vi "mw-dar.vi"() -> ()   [LabVIEW 2022 SP3]
panel:
  in  "Stopp":bool
  out "Zählung Speicherwerte":dbl
  out "Speichervorgang läuft":bool
  in  "Start Datenspeicherung":bool
  in  "Anzahl Messerte zum speichern":dbl
  out "Maximalwert Kurve 3":dbl format="%#.2g"
  out "Minimalwert Kurve 3":dbl format="%#.2g"
  out "Minimalwert Kurve 2":dbl format="%#.2g"
  out "Maximalwert Kurve 2":dbl format="%#.2g"
  out "niedriger Kurve 3":bool
  out "hoeher Kurve 3":bool
  out "niedriger Kurve 2":bool
  out "hoeher Kurve 2":bool
  out "Zufalszahl Kurve 2":dbl
  out "Zufalszahl Kurve 3":dbl
  out "hoeher Kurve 1":bool
  out "Maximalwert Kurve 1":dbl format="%#.2g"
  out "Zufalszahl Kurve 1":dbl
  out "Minimalwert Kurve 1":dbl format="%#.2g"
  out "niedriger Kurve 1":bool
  out "Anzahl Messwerte":dbl
  out "Kurvenverläufe":T1(graph)
  # "Aktuelle Werte"
  # "Minimale Werte"
  # "Maximale Werte"
  # "Kurve 1"
  # "Kurve 2"
  # "Kurve 3"
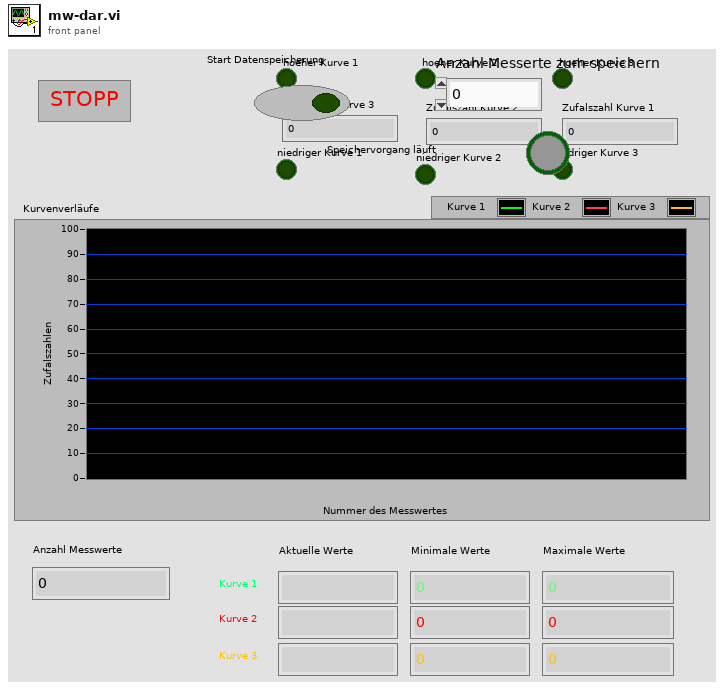
[diagram p1: front panel]
types:
  T1 = cluster{"Zufalszahl":dbl, "Zufalszahl":dbl, "Zufalszahl":dbl}
  T2 = cluster{"Zufalszahl":dbl, "Zufalszahl":dbl, "Zufalszahl":dbl}[]
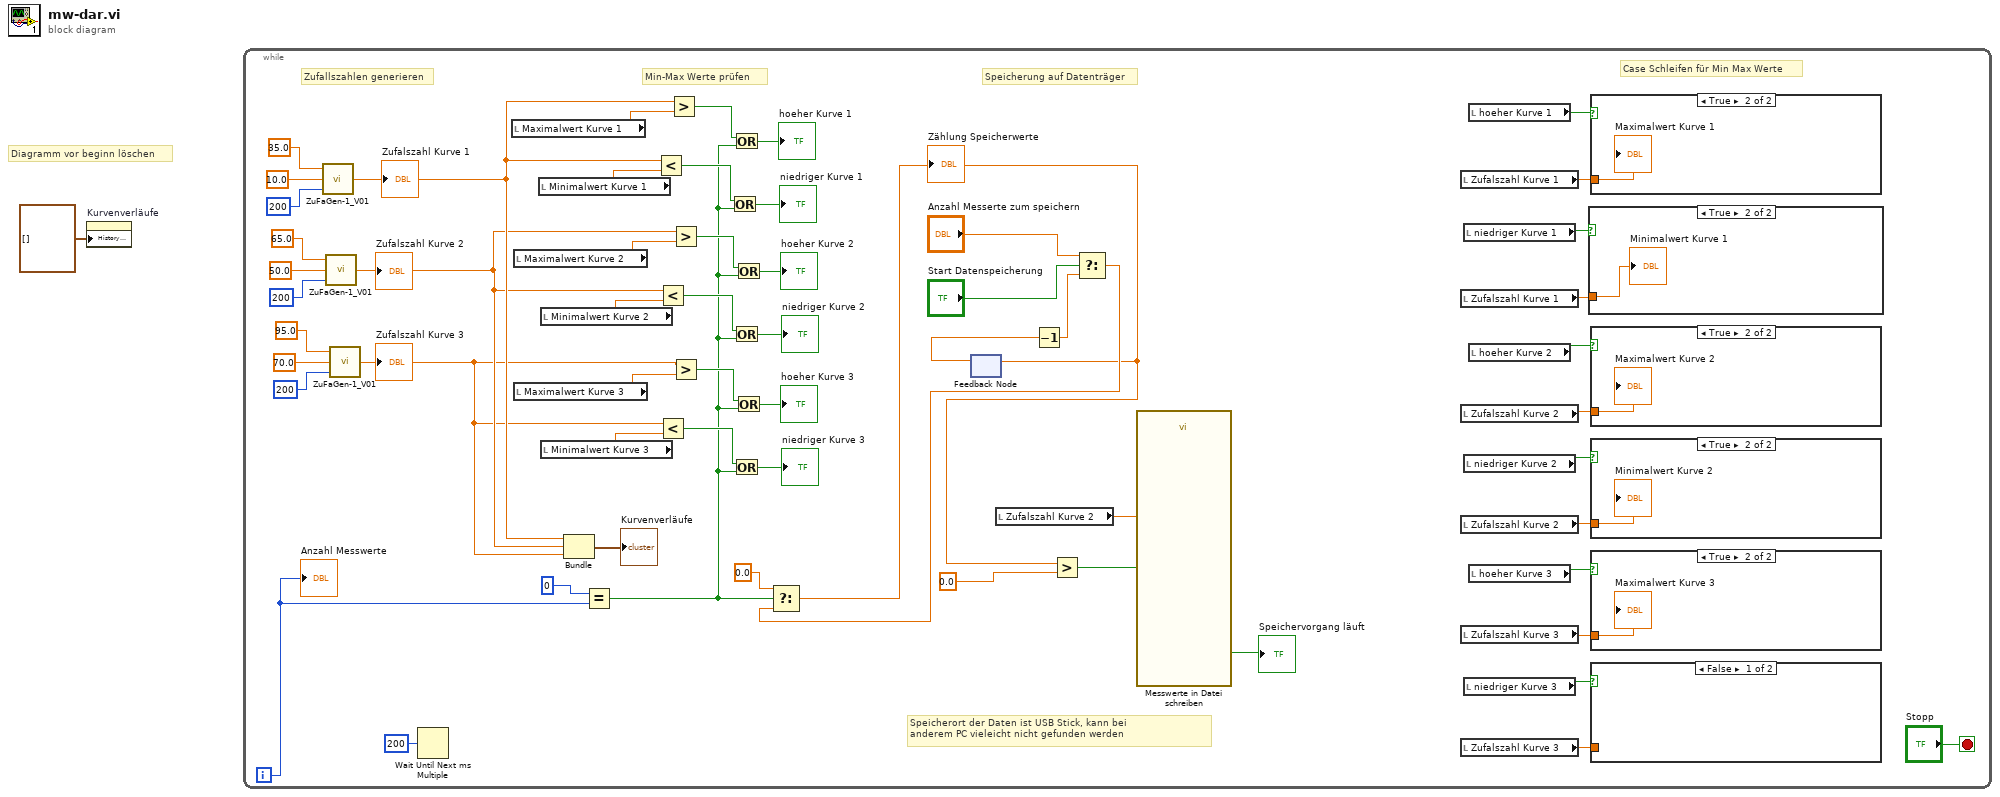
[diagram p0: block diagram]
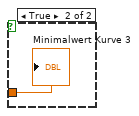
[diagram p2: hidden frame]
diagram:
  # "Diagramm vor beginn löschen"
  n1 = property on="Kurvenverläufe" class="WFChart (strict)"("History Data"=T2 [] ("Historiendaten")) -> ()  [unwired: 2 in, 2 out]
  n2 = while {
    i -> [w49]
    stop <- "Stopp" stop-if-true
    # "Speicherung auf Datenträger"
    # "Min-Max Werte prüfen"
    # "Case Schleifen für Min Max Werte"
    # "Speicherort der Daten ist USB Stick, kann bei \nanderem PC vieleicht nicht gefunden werden"
    # "Zufallszahlen generieren"
    n3 = call "ZuFaGen-1_V01.vi"("Zeitlicher Abstand / ms"=u32 200, "Untre Grenze"=10.0, "Obere Grenze"=35.0) -> ("Zufalszahl"=w41:dbl)
    "Zufalszahl Kurve 1" <- w41
    n4 = call "ZuFaGen-1_V01.vi"("Zeitlicher Abstand / ms"=u32 200, "Untre Grenze"=50.0, "Obere Grenze"=65.0) -> ("Zufalszahl"=w28:dbl)
    "Zufalszahl Kurve 2" <- w28
    n5 = call "ZuFaGen-1_V01.vi"("Zeitlicher Abstand / ms"=u32 200, "Untre Grenze"=70.0, "Obere Grenze"=95.0) -> ("Zufalszahl"=w27:dbl)
    "Zufalszahl Kurve 3" <- w27
    n6 = Wait Until Next ms Multiple(millisecond multiple=u32 200 ("ms")) -> ()  [unwired: 1 out]
    n7 = local read "Maximalwert Kurve 1"() -> (w43:dbl)
    n8 = local read "Maximalwert Kurve 2"() -> (w39:dbl)
    n9 = local read "Maximalwert Kurve 3"() -> (w30:dbl)
    n10 = local read "Minimalwert Kurve 1"() -> (w42:dbl)
    n11 = local read "Minimalwert Kurve 2"() -> (w40:dbl)
    n12 = local read "Minimalwert Kurve 3"() -> (w29:dbl)
    n13 = Bundle ("Bündeln")("Zufalszahl"=w41, "Zufalszahl"=w28, "Zufalszahl"=w27) -> (→"Kurvenverläufe":T1)  [unwired: 1 in]
    n14 = Equal?(x=0, y=w49) -> (x = y?=w6:bool)
    n15 = Less?(x=w41, y=w42) -> (x < y?=w45:bool)
    n16 = Less?(x=w28, y=w40) -> (x < y?=w37:bool)
    n17 = Less?(x=w27, y=w29) -> (x < y?=w32:bool)
    n18 = Greater?(x=w41, y=w43) -> (0:w44:bool)
    n19 = Greater?(x=w28, y=w39) -> (0:w38:bool)
    n20 = Greater?(x=w27, y=w30) -> (0:w31:bool)
    n21 = Or(x=w45, y=w6) -> (x .or. y?=→"niedriger Kurve 1":bool)
    n22 = Or(x=w44, y=w6) -> (x .or. y?=→"hoeher Kurve 1":bool)
    n23 = Or(x=w37, y=w6) -> (x .or. y?=→"niedriger Kurve 2":bool)
    n24 = Or(x=w32, y=w6) -> (x .or. y?=→"niedriger Kurve 3":bool)
    n25 = Or(x=w38, y=w6) -> (x .or. y?=→"hoeher Kurve 2":bool)
    n26 = Or(x=w31, y=w6) -> (x .or. y?=→"hoeher Kurve 3":bool)
    n27 = feedback #1 ("Rückkopplungsknoten")() -> (w23:dbl)  [unwired: 1 in]
    n28 = local read "Zufalszahl Kurve 2"() -> (w25:dbl)
    n29 = Decrement(x=w23) -> (x-1=w21:dbl)
    n30 = Select(t="Anzahl Messerte zum speichern", s="Start Datenspeicherung", f=w21) -> (s? t:f=w4:dbl)
    n31 = Select(t=0.0, s=w6, f=w4) -> (s? t:f=w2:dbl)
    "Zählung Speicherwerte" <- w2
    n32 = feedback-in #1(w2) -> ()
    n33 = Greater?(x=w2, y=0.0) -> (0:w24:bool)
    n34 = call "Messwerte in Datei schreiben"("Signals"=w25, "Enable"=w24) -> ("Saving Data"=→"Speichervorgang läuft":bool)  [unwired: 15 in, 2 out]
    n35 = local read "Zufalszahl Kurve 1"() -> (w19:dbl)
    n36 = local read "Zufalszahl Kurve 1"() -> (w17:dbl)
    n37 = local read "Zufalszahl Kurve 2"() -> (w14:dbl)
    n38 = local read "Zufalszahl Kurve 2"() -> (w13:dbl)
    n39 = local read "Zufalszahl Kurve 3"() -> (w11:dbl)
    n40 = local read "Zufalszahl Kurve 3"() -> (w7:dbl)
    n41 = local read "niedriger Kurve 1"() -> (w16:bool)
    n42 = local read "niedriger Kurve 2"() -> (w12:bool)
    n43 = local read "niedriger Kurve 3"() -> (w8:bool)
    n44 = local read "hoeher Kurve 1"() -> (w18:bool)
    n45 = local read "hoeher Kurve 2"() -> (w15:bool)
    n46 = local read "hoeher Kurve 3"() -> (w10:bool)
    n47 = case shown="True" w16 {
      tunnel: w17 -> [_ w65]
      frame False {
      }
      frame True {
        "Minimalwert Kurve 1" <- w65
      }
    }
    n48 = case shown="True" w18 {
      tunnel: w19 -> [_ w66]
      frame False {
      }
      frame True {
        "Maximalwert Kurve 1" <- w66
      }
    }
    n49 = case shown="True" w15 {
      tunnel: w14 -> [_ w64]
      frame False {
      }
      frame True {
        "Maximalwert Kurve 2" <- w64
      }
    }
    n50 = case shown="True" w12 {
      tunnel: w13 -> [_ w63]
      frame False {
      }
      frame True {
        "Minimalwert Kurve 2" <- w63
      }
    }
    n51 = case shown="True" w10 {
      tunnel: w11 -> [_ w62]
      frame False {
      }
      frame True {
        "Maximalwert Kurve 3" <- w62
      }
    }
    n52 = case shown="False" w8 {
      tunnel: w7 -> [_ w61]
      frame False {
      }
      frame True {
        "Minimalwert Kurve 3" <- w61
      }
    }
    "Anzahl Messwerte" <- w49
  }
